vi "set_params.vi"(0 "_stage in":refnum<class "_stage.lvclass">, 3 "error in (no error)":errorcluster) -> (7 "_stage out":refnum<class "_stage.lvclass">, 10 "error out":errorcluster)   [LabVIEW 2019, in "_stage.lvlib" / "_stage.lvclass"]
uses:
  _stage.lvclass
panel:
  in  "OK Button":bool
  in  "pos_max":dbl[](array[numeric])
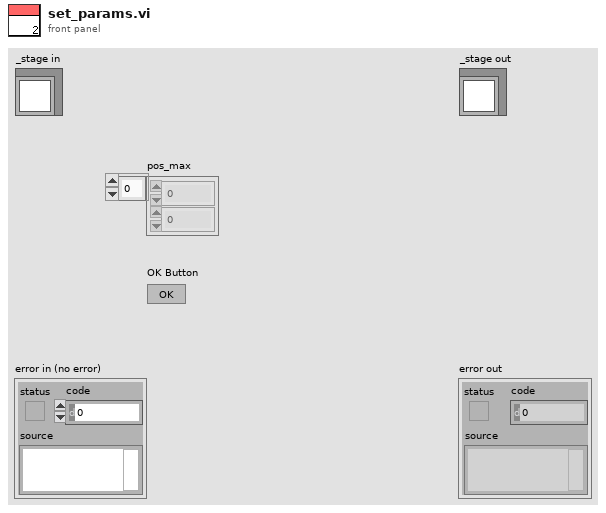
[diagram p1: front panel]
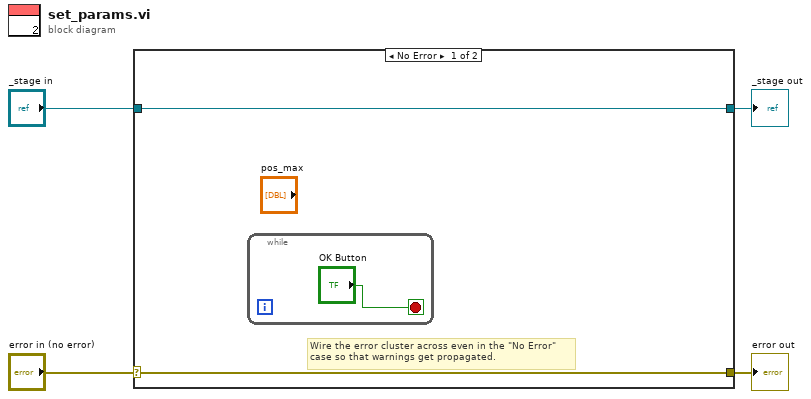
[diagram p0: block diagram]
diagram:
  n1 = case shown="No Error" "error in (no error)" {
    selector: "error in (no error)" -> [w6 w9]
    tunnel: [w6 w9] -> w3
    tunnel: [w5 w8] -> w1
    tunnel: "_stage in" -> [w5 w8]
    frame No Error {
      # "Wire the error cluster across even in the \"No Error\"\ncase so that warnings get propagated."
      n2 = while {
        stop <- "OK Button" stop-if-true
      }
    }
    frame Error {
    }
  }
  "error out" <- w3
  "_stage out" <- w1
